vi "LL_BuildElementPath_StringArray.vi"(10 "Names":string[](array[string]), 11 "parent Name":string) -> (3 "full name":string[](array[string]))   [LabVIEW 2017, in "TOML.lvlib"]
uses:
  TOML.lvlib
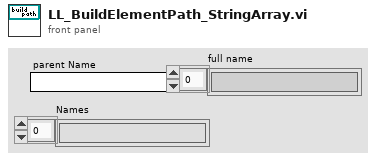
[diagram p1: front panel]
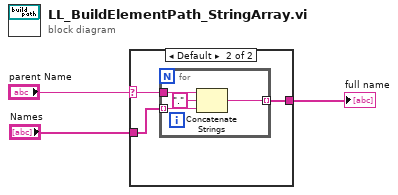
[diagram p0: block diagram]
diagram:
  n1 = case shown="Default" "parent Name" {
    selector: "parent Name" -> [_ w5]
    tunnel: [w4 w7] -> w3
    tunnel: "Names" -> [w4 w6]
    frame "" {
    }
    frame Default {
      n2 = for {
        tunnel: [w10] -> w7 mode=indexing
        tunnel: w6 -> [w9] mode=indexing
        tunnel: w5 -> [w8]
        n3 = Concatenate Strings(w8, "." ("string"), w9) -> (w10:string)
      }
    }
  }
  "full name" <- w3
